vi "Draw Filled Rect.vi"(6 "Left":bool, 8 "Limits":dbl[](array[numeric]), 9 "Scores":dbl[](array[numeric]), 10 "Bounding Box":T2, 11 "image in":T1) -> (3 "image out":T1)   [LabVIEW 2013]
doc: "Add a rectangle border around the inside and outside of what is believed to be the reflective tape. Also place the color coded scores next to all of the large blobs being processed."
uses:
  <vilib>/vision/Image Controls.llb/IMAQ Image.ctl
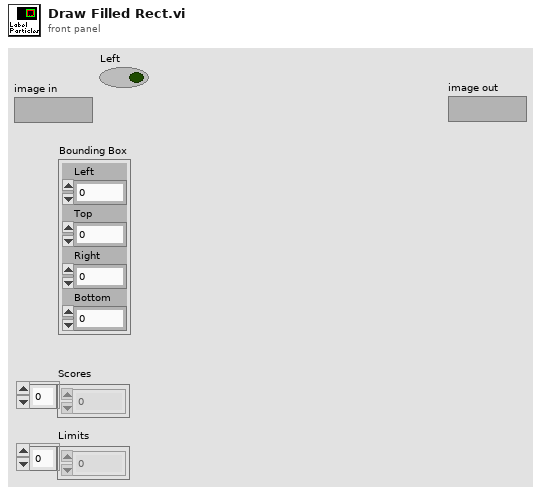
[diagram p1: front panel]
types:
  T1 = typedef "IMAQ Image.ctl" = refnum<image>
  T2 = cluster{"Left":dbl, "Top":dbl, "Right":dbl, "Bottom":dbl}
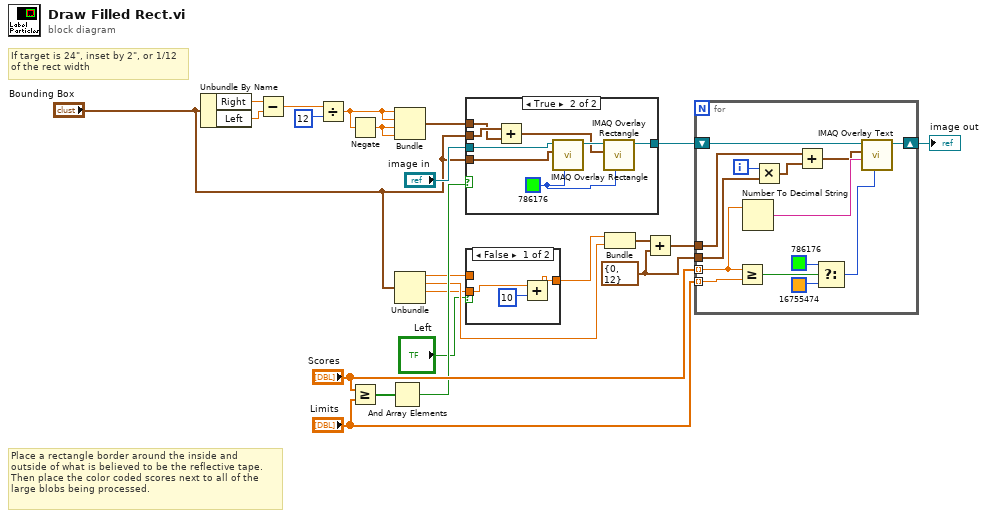
[diagram p0: block diagram]
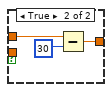
[diagram p2: hidden frame]
diagram:
  w10 = cluster{i32, i32} {0, 12}
  # "Place a rectangle border around the inside and\noutside of what is believed to be the reflective tape.\nThen place the color coded scores next to all of the\nlarge blobs being processed."
  # "If target is 24\", inset by 2\", or 1/12\nof the rect width"
  n1 = Unbundle By Name("Bounding Box") -> ("Right"=w8:dbl, "Left"=w7:dbl)
  n2 = Subtract(x=w8, y=w7) -> (x-y=w5:dbl)
  n3 = Divide(x=w5, y=12) -> (x/y=w3:dbl)
  n4 = Negate(x=w3) -> (-x=w9:dbl)
  n5 = Greater Or Equal?(x="Scores", y="Limits") -> (x >= y?=w21:bool[])
  n6 = And Array Elements(Boolean array=w21) -> (logical AND=w18:bool)
  n7 = Bundle(w3, w3, w9, w9) -> (w6:cluster{dbl, dbl, dbl, dbl})  [unwired: 1 in]
  n8 = Unbundle("Bounding Box") -> ("Left"=w14:dbl, "Top"=w15:dbl, "Right"=w1:dbl)  [unwired: 1 out]
  n9 = case shown="True" w18 {
    tunnel: "image in" -> [w24 w32]
    tunnel: "Bounding Box" -> [_ w31]
    tunnel: "Bounding Box" -> [_ w29]
    tunnel: [w24 w27] -> w16
    tunnel: w6 -> [_ w25]
    frame False {
    }
    frame True {
      w26 = u32 786176 ("Color")
      n10 = Add(x=w29, y=w25) -> (x+y=w28:cluster{dbl, dbl, dbl, dbl})
      n11 = call "IMAQ Overlay Rectangle"("Color"=w26, "Rectangle"=w31, "Image"=w32) -> ("Image Out"=w30:T1)  [unwired: 3 in, 5 out]
      n12 = call "IMAQ Overlay Rectangle"("Color"=w26, "Rectangle"=w28, "Image"=w30) -> ("Image Out"=w27:T1)  [unwired: 3 in, 5 out]
    }
  }
  n13 = case shown="False" "Left" {
    tunnel: w14 -> [_ w38]
    tunnel: [w34 w37] -> w13
    tunnel: w1 -> [w33 _]
    frame False {
      n14 = Add(x=w33, y=10) -> (x+y=w34:dbl)
    }
    frame True {
      n15 = Subtract(x=w38, y=30) -> (x-y=w37:dbl)
    }
  }
  n16 = Bundle(w13, "Top"=w15) -> (w12:cluster{dbl, "Top":dbl})  [unwired: 1 in]
  n17 = Add(x=w12, y=w10) -> (x+y=w11:cluster{dbl, dbl})
  n18 = for {
    shift-right: [w51] -> w22
    shift-left: w16 -> [w52]
    tunnel: "Scores" -> [w44] mode=indexing
    tunnel: "Limits" -> [w50] mode=indexing
    tunnel: w10 -> [w41]
    tunnel: w11 -> [w40]
    i -> [w43]
    n19 = Greater Or Equal?(x=w44, y=w50) -> (x >= y?=w49:bool)
    n20 = Number To Decimal String(number=w44) -> (decimal integer string=w46:string)  [unwired: 1 in]
    n21 = Multiply(x=w43, y=w41) -> (x*y=w42:cluster{i32, i32})
    n22 = Add(x=w40, y=w42) -> (x+y=w39:cluster{dbl, dbl})
    n23 = Select(t=u32 786176 ("Color"), s=w49, f=u32 16755474 ("Color")) -> (s? t:f=w45:u32)
    n24 = call "IMAQ Overlay Text"("Text Color (black)"=w45, "String"=w46, "Origin"=w39, "Image"=w52) -> ("Image Out"=w51:T1)  [unwired: 6 in, 1 out]
  }
  "image out" <- w22
